vi "Run Custom Device Post Initialization VI.vi"(8 "error in (no error)":errorcluster, 9 "Custom Device Ref":T1, 10 "Settings":T2(array[cluster]), 11 "Post Initialization VI":path) -> (0 "error out":errorcluster)   [LabVIEW 2019, in "Simple SysDef API.lvlib"]
uses:
  <userlib>/SimpleSysDef/Simple SysDef API.lvlib
  <userlib>/SimpleSysDef/_SubVIs/Custom Device Control Name and Ref.ctl
  NationalInstruments.VeriStand.SystemDefinitionAPI
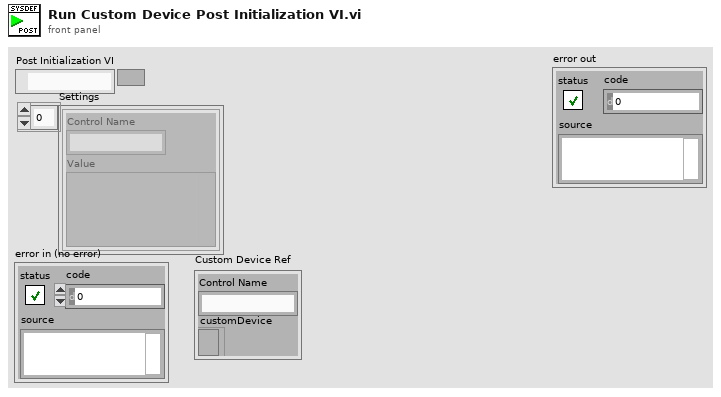
[diagram p1: front panel]
types:
  T1 = typedef "Simple SysDef API.lvlib/Custom Device Control Name and Ref.ctl" = cluster{"customDevice":refnum<k24>, "Control Name":string}
  T2 = cluster{"Control Name":string, "Value":variant}[]
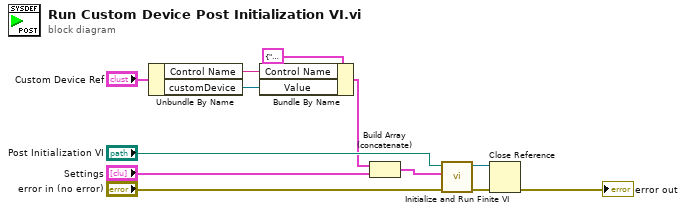
[diagram p0: block diagram]
diagram:
  n1 = Unbundle By Name("Custom Device Ref") -> ("Control Name"=w3:string, "customDevice"=w2:refnum<k24>)
  n2 = Bundle By Name(cluster=cluster{"Control Name":string, "Value":variant} {"Control Name"="", "Value"=variant}, "Control Name"=w3, "Value"=w2) -> (w1:cluster{"Control Name":string, "Value":variant})
  n3 = Build Array (concatenate)(w1, "Settings") -> (w6:T2)
  n4 = call <userlib>:"Initialize and Run Finite VI.vi"("error in (no error)"="error in (no error)", "Settings"=w6, "Initialization VI"="Post Initialization VI") -> ("error out"=w9:errorcluster, "VI out"=w8:refnum<vi>)  [unwired: 7 in]
  n5 = Close Reference(reference=w8, error in (no error)=w9) -> (error out=→"error out":errorcluster)
